vi "testRSAEncrypt&DecryptNoData.vi"(8 "error in (no error)":errorcluster, 11 "TestCase in":refnum<class "TestRSA.lvclass">) -> (0 "error out":errorcluster, 3 "TestCase out":refnum<class "TestRSA.lvclass">)   [LabVIEW 2021, in "TestRSA.lvclass"]
uses:
  TestRSA.lvclass
  Asymmetric Encryption/RSA/RSAEncryptionPadding.ctl
  TestRSA.lvclass/TestRSA.ctl
  <vilib>/addons/_JKI Toolkits/VI Tester/TestCase.llb/TestCase.lvclass
  Asymmetric Encryption/dotNET Crypto Asymmetric Encryption.lvlib
  Key Management/dotNET Crypto Key Management.lvlib
  C:/Program Files (x86)/National Instruments/LabVIEW 2021/vi.lib/addons/_JKI Toolkits/VI Tester/TestCase.llb/TestCase.lvclass
panel:
  out "Decrypted data":string
  out "Encrypted data":string
  out "Encrypted data out":u8[](array[numeric])
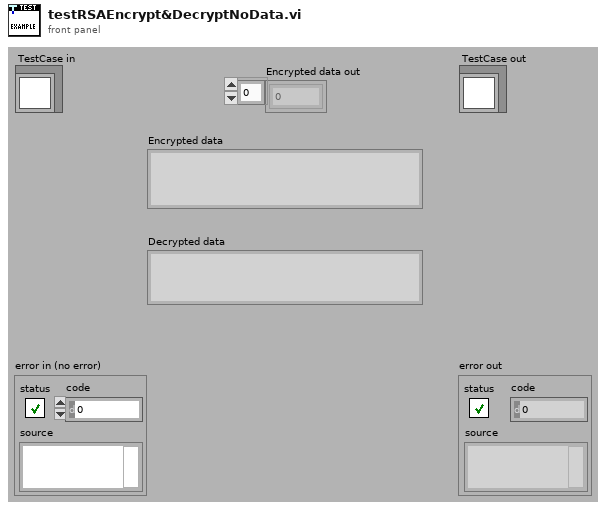
[diagram p1: front panel]
types:
  T1 = typedef "dotNET Crypto Asymmetric Encryption.lvlib/RSAEncryptionPadding.ctl" = enum16{"OaepSHA1", "OaepSHA256", "OaepSHA384", "OaepSHA512", "Pkcs1"}
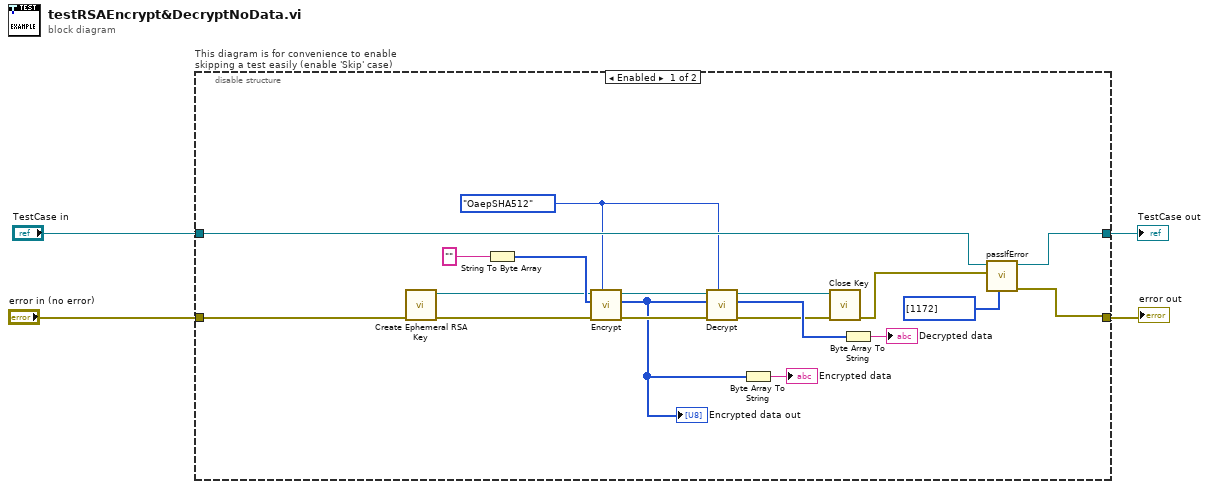
[diagram p0: block diagram]
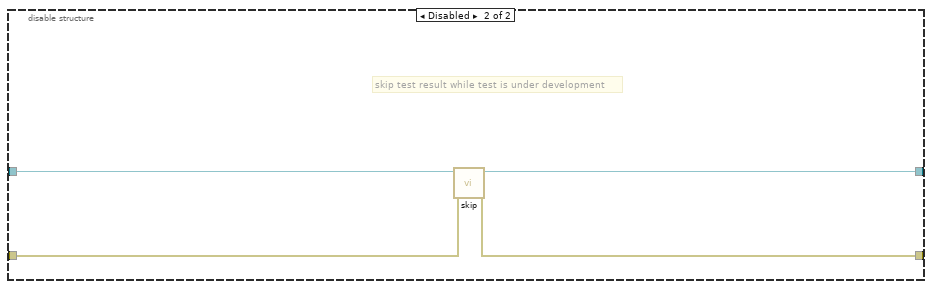
[diagram p2: hidden frame]
diagram:
  n1 = disable-structure "This diagram is for convenience to enable skipping a test easily (enable 'Skip' case)" shown="Enabled" {
    disable-tunnel: "TestCase in" -> [w23 w27]
    disable-tunnel: [w22 w25] -> w1
    disable-tunnel: [w21 w26] -> w3
    disable-tunnel: "error in (no error)" -> [w7 w24]
    frame Enabled {
      w19 = RSAEncryptionPadding."OaepSHA512" ("Padding Mode")
      n2 = call "Create Ephemeral RSA Key.vi"("error in (no error)"=w7) -> ("error out"=w6:errorcluster, "CngKey out"=w5:refnum<k24>)  [unwired: 9 in]
      n3 = String To Byte Array(string="") -> (unsigned byte array=w13:u8[])
      n4 = call "Encrypt.vi"("Padding Mode"=w19, "error in (no error)"=w6, "Raw data in"=w13, "CngKey in"=w5) -> ("error out"=w20:errorcluster, "Encrypted data out"=w12:u8[], "CngKey out"=w17:refnum<k24>)  [unwired: 5 in]
      "Encrypted data out" <- w12
      n5 = call "Decrypt.vi"("Padding Mode"=w19, "error in (no error)"=w20, "Encrypted data in"=w12, "CngKey in"=w17) -> ("error out"=w10:errorcluster, "Raw data out"=w11:u8[], "CngKey out"=w8:refnum<k24>)  [unwired: 5 in]
      n6 = Byte Array To String(unsigned byte array=w12) -> (string=→"Encrypted data":string)
      n7 = call "Close Key.vi"("error in (no error)"=w10, "CngKey in"=w8) -> ("error out"=w9:errorcluster)  [unwired: 9 in]
      n8 = Byte Array To String(unsigned byte array=w11) -> (string=→"Decrypted data":string)
      n9 = call-dynamic "passIfError.vi"("passing error codes (default = any error code)"=i32[] [1172], "error"=w9, "TestCase in"=w23) -> ("error out"=w21:errorcluster, "TestCase out"=w22:refnum<class "TestRSA.lvclass">)  [unwired: 7 in]
    }
    frame Disabled {
      # "skip test result while test is under development"
      n10 = call <vilib>:"skip.vi"("error in (no error)"=w24, "TestCase in"=w27) -> ("error out"=w26:errorcluster, "TestCase out"=w25:refnum<class "TestRSA.lvclass">)  [unwired: 8 in]
    }
  }
  "error out" <- w3
  "TestCase out" <- w1
